vi "OptionalCameraCalib.vi"(8 "error in":errorcluster) -> (0 "PixUmConversion":ext, 1 "WorkingDistance":ext, 2 "RunCameraCalibration":bool=TRUE, 3 "error out":errorcluster)   [LabVIEW 2016]
uses:
  <vilib>/regexp/Match Regular Expression.xnode
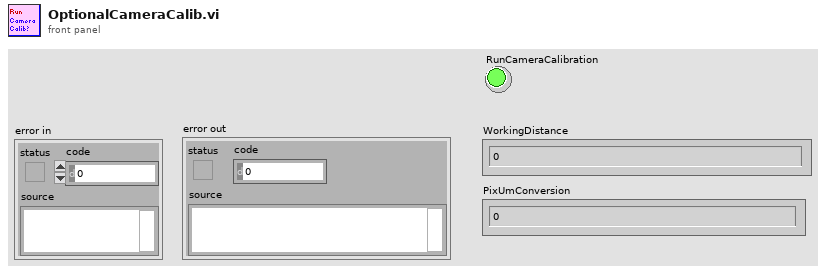
[diagram p1: front panel]
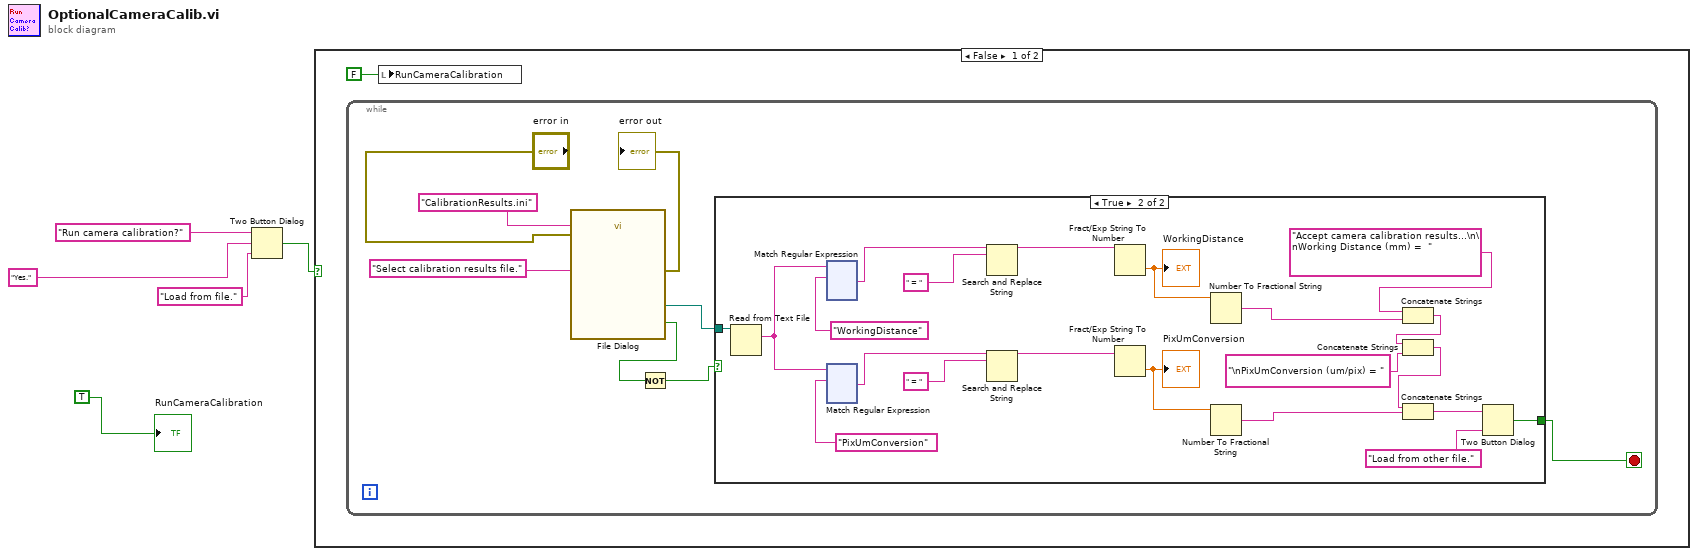
[diagram p0: block diagram]
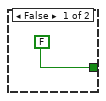
[diagram p2: hidden frame]
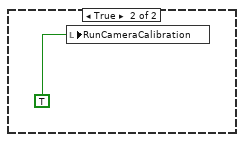
[diagram p3: hidden frame]
diagram:
  n1 = Two Button Dialog(message="Run camera calibration?", 1:"Load from file." ("F button name (\"Cancel\")"), 2:"Yes." ("T button name (\"OK\")")) -> (T button?=w2:bool)
  n2 = case shown="False" w2 {
    frame False {
      n3 = while {
        stop <- w11 stop-if-true
        n4 = call "File Dialog"("prompt"="Select calibration results file.", "default name"="CalibrationResults.ini", "error in"="error in") -> ("selected path"=w12:path, "cancelled"=w10:bool, "error out"=→"error out":errorcluster)  [unwired: 9 in, 1 out]
        n5 = Not(x=w10) -> (.not. x?=w9:bool)
        n6 = case shown="True" w9 {
          tunnel: w12 -> [_ w36]
          tunnel: [FALSE w20] -> w11
          frame False {
          }
          frame True {
            n7 = Read from Text File(file (use dialog)=w36) -> (text=w35:string)  [unwired: 3 in, 3 out]
            n8 = xnode "Match Regular Expression"("input string"=w35, "regular expression"="WorkingDistance") -> ("after match"=w32:string)  [unwired: 4 in, 4 out]
            n9 = xnode "Match Regular Expression"("input string"=w35, "regular expression"="PixUmConversion") -> ("after match"=w30:string)  [unwired: 4 in, 4 out]
            n10 = Search and Replace String(input string=w32, search string=" = ") -> (result string=w28:string)  [unwired: 6 in, 3 out]
            n11 = Search and Replace String(input string=w30, search string=" = ") -> (result string=w23:string)  [unwired: 6 in, 3 out]
            n12 = Fract/Exp String To Number(string=w28) -> (number=w19:dbl)  [unwired: 3 in, 1 out]
            "WorkingDistance" <- w19
            n13 = Fract/Exp String To Number(string=w23) -> (number=w17:dbl)  [unwired: 3 in, 1 out]
            "PixUmConversion" <- w17
            n14 = Number To Fractional String(number=w19) -> (F-format string=w18:string)  [unwired: 3 in]
            n15 = Number To Fractional String(number=w17) -> (F-format string=w16:string)  [unwired: 3 in]
            n16 = Concatenate Strings("Accept camera calibration results...\n\nWorking Distance (mm) =  " ("string"), w18) -> (w26:string)
            n17 = Concatenate Strings(w26, "\nPixUmConversion (um/pix) = " ("string")) -> (w24:string)
            n18 = Concatenate Strings(w24, w16) -> (w22:string)
            n19 = Two Button Dialog(message=w22, 1:"Load from other file." ("F button name (\"Cancel\")")) -> (T button?=w20:bool)  [unwired: 1 in]
          }
        }
      }
      n20 = local write "RunCameraCalibration"(FALSE ("RunCameraCalibration")) -> ()
    }
    frame True {
      n21 = local write "RunCameraCalibration"(TRUE ("RunCameraCalibration")) -> ()
    }
  }
  "RunCameraCalibration" <- TRUE
